vi "Apply Limits.vi"(8 "error in":errorcluster, 11 "6032A in":refnum<class "6032A.lvclass">) -> (0 "error out":errorcluster, 3 "6032A out":refnum<class "6032A.lvclass">)   [LabVIEW 2019, in "6032A.lvlib" / "6032A.lvclass"]
uses:
  Library/6032A.lvclass
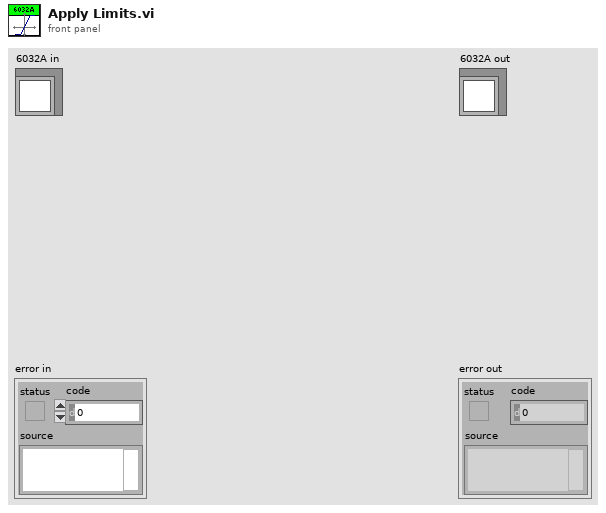
[diagram p1: front panel]
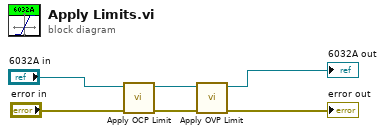
[diagram p0: block diagram]
diagram:
  n1 = call "Apply OCP Limit.vi"("error in"="error in", "6032A in"="6032A in") -> ("error out"=w6:errorcluster, "6032A out"=w3:refnum<class "6032A.lvclass">)  [unwired: 8 in]
  n2 = call "Apply OVP Limit.vi"("error in"=w6, "6032A in"=w3) -> ("error out"=→"error out":errorcluster, "6032A out"=→"6032A out":refnum<class "6032A.lvclass">)  [unwired: 8 in]
